vi "Motor_pwm_controle_de_posicao_3.vi"() -> ()   [LabVIEW 2018]
uses:
  <vilib>/Platform/TimedLoop/XDataNode/timing_clust.ctl
  <vilib>/Platform/TimedLoop/XDataNode/nitl_modes.ctl
  <vilib>/Platform/TimedLoop/XDataNode/wakeup.ctl
  <vilib>/Analysis/3filter.llb/Savitzky-Golay Filter (DBL).vi
  <vilib>/platform/TimedLoop/XDataNode/XDataNode.xnode
  <vilib>/Platform/TimedLoop/XDataNode/XDNodeRunTimeDep.lvlib
  <vilib>/Analysis/NI_AALBase.lvlib
panel:
  out "size(s)":i32
  out "Posições alcançadas (°)":dbl[](array[numeric])
  in  "Posições desejadas (°)":dbl[](array[numeric])
  out "Posição do motor":dbl[](graph)
  out "Aceleração":dbl[](graph)
  out "Velocidade de rotação do motor":dbl[](graph)
  out "Diferença entre a posição atual e a desejada (°)":dbl
  in  "Taxa de convergência":dbl(slide) scale=0.0..5.0
  out "Sentido de Rotação":enum16{"Horário", "Anti-Horário"}(ring)
  in  "Tab Control":enum32{"Posição", "Velocidade", "Aceleração"}(tab)
  out "Posição Acumulada":waveform(dbl)(graph)
  out "Velocidade Acumulada":waveform(dbl)(graph)
  out "Aceleração acumulada":waveform(dbl)(graph)
  in  "Frequência do PWM (Hz)":dbl
  in  "stop":bool
  in  "Iniciar controle":bool
  in  "Tensão de alimentação (V)":dbl
  # "CONTROLE DE POSI敲O DE MOTOR DC"
  # "Controle de posição por PWM desenvolvido para um motor DC simulado"
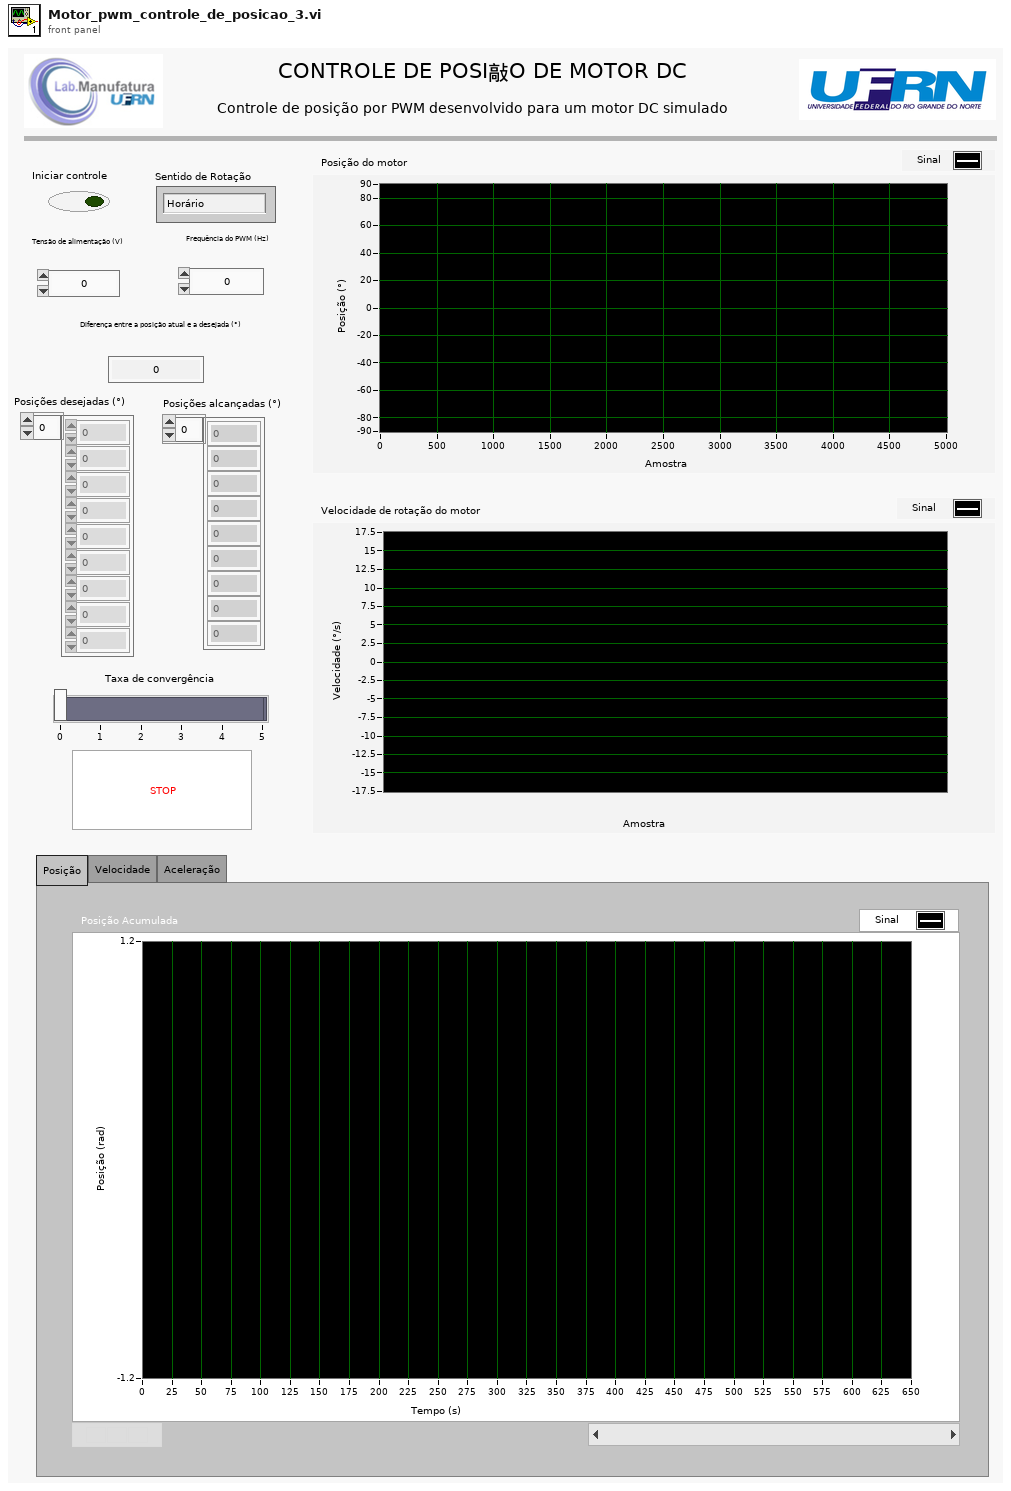
[diagram p1: front panel]
types:
  T1 = typedef "XDNodeRunTimeDep.lvlib/timing_clust.ctl" = cluster{"Expected End [f-1]":u64, "Actual End [f-1]":u64, "Finished Late? [f-1]":bool, "Expected End [i-1]":u64, "Actual End [i-1]":u64, "Finished Late? [i-1]":bool, "Expected Start [i]":u64, "Actual Start [i]":u64, "Expected Start [f]":u64, "Actual Start [f]":u64, "Source Name":string, "Structure Name":string, "Period":i64, "Deadline":i64, "Offset":i64, "Start":i64, "Priority":i32, "Timeout":i32, "Mode":T2, "Wakeup Reason":T3, "Error":errorcluster, "Source Type":string, "Secondary Source Type":string, "Global End Time":u64, "Global Start Time":u64, "Frame Duration":u64, "Iteration Duration":u64, "Assigned CPU":i32, "I/O Scan Engine Mode":u32}
  T2 = typedef "XDNodeRunTimeDep.lvlib/nitl_modes.ctl" = enum32{"No Change", "Process missed periods, maintain original phase", "Discard missed periods, maintain original phase", "Process missed periods, ignore original phase", "Discard missed periods, ignore original phase"}
  T3 = typedef "XDNodeRunTimeDep.lvlib/wakeup.ctl" = enum32{"Normal", "Aborted", "Asynchronous wakeup", "Timing source error", "Timed loop error", "Timeout"}
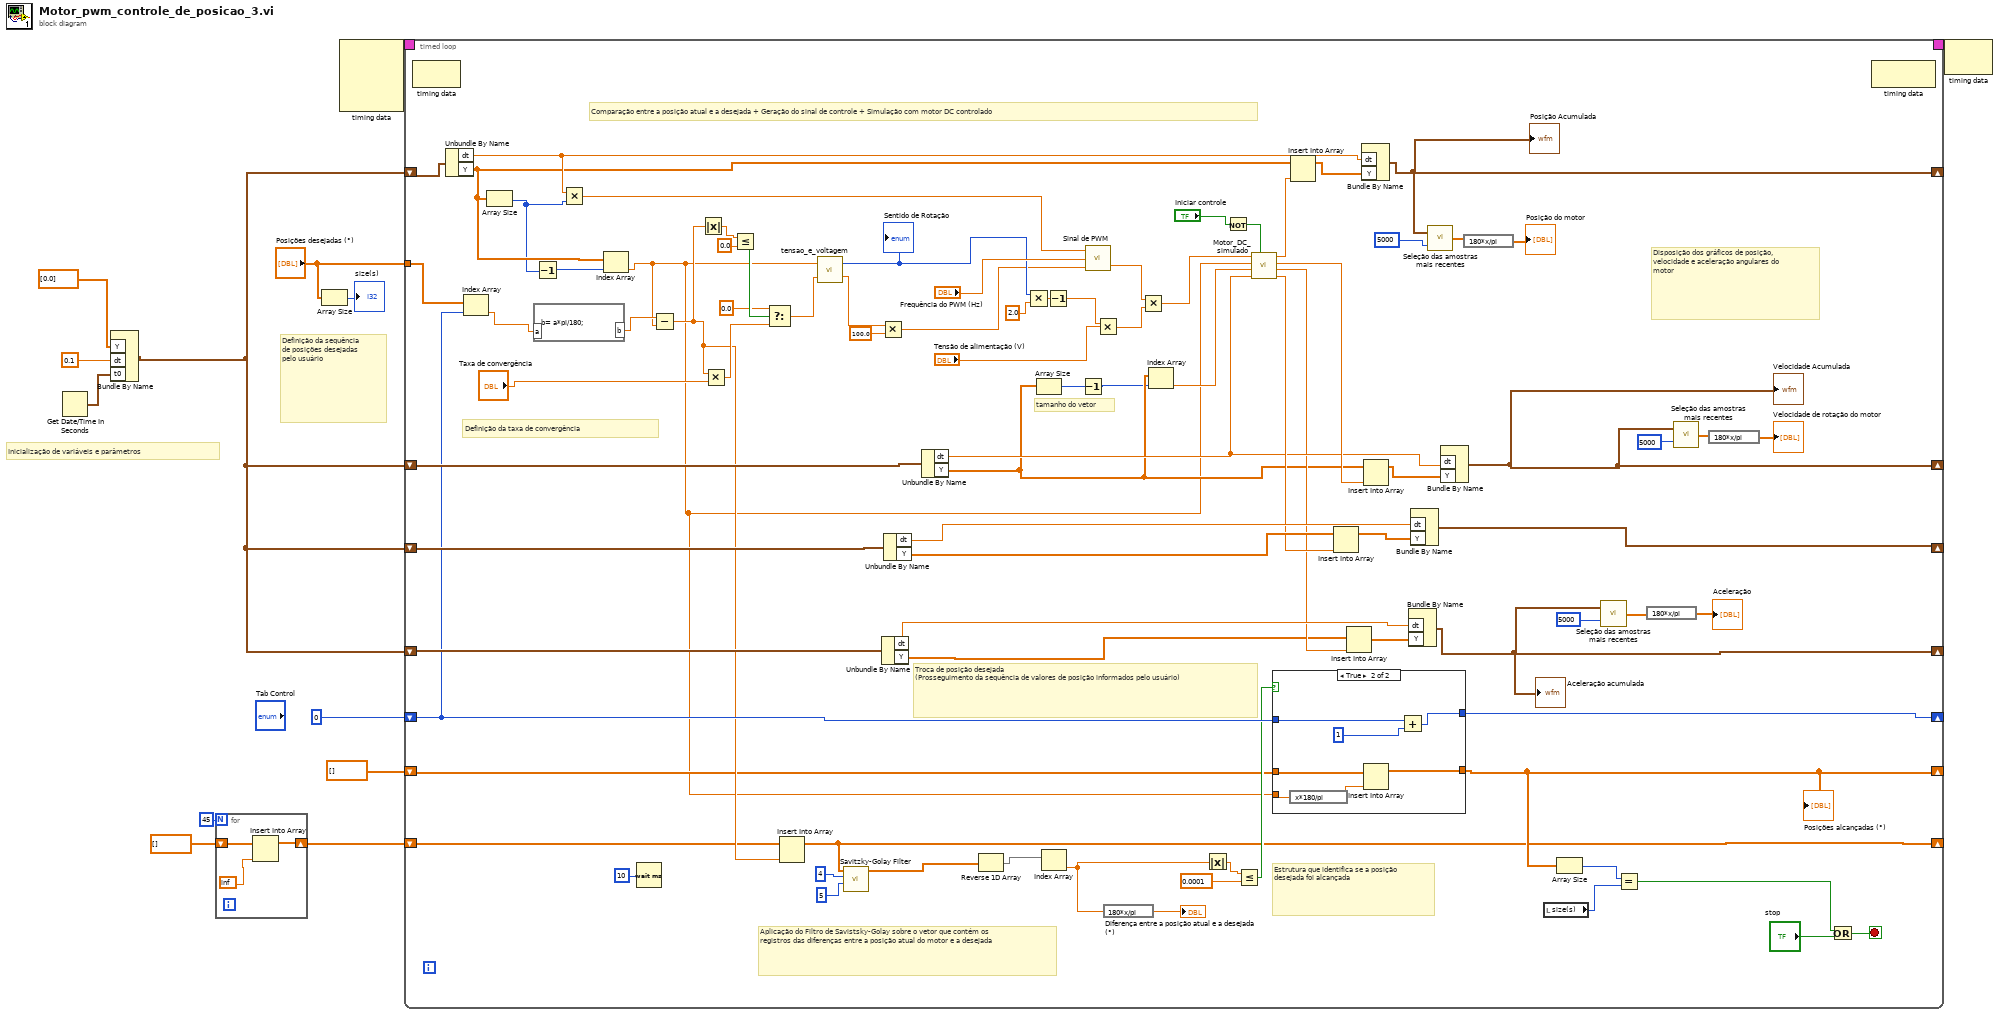
[diagram p0: block diagram]
diagram:
  # "Inicialização de variáveis e parâmetros"
  # "Definição da sequência de posições desejadas pelo usuário"
  n1 = Get Date/Time In Seconds() -> (seconds since 1Jan1904=w10:timestamp)
  n2 = Bundle By Name("Y"=dbl[] [0.0], "dt"=0.1, "t0"=w10) -> (w8:waveform(dbl))  [unwired: 1 in]
  n3 = for {
    N: 45 -> [_]
    shift-right: [w15] -> w4
    shift-left: dbl[] [] ("array") -> [w16]
    n4 = Insert Into Array(array=w16, new element=inf ("new element/subarray")) -> (w15:dbl[])  [unwired: 1 in]
  }
  n5 = Array Size(array="Posições desejadas (°)") -> (size(s)=→"size(s)":i32)
  n6 = node-c288() -> (w13:T1)  [unwired: 4 in]
  n7 = timed-loop {
    shift-right: [w99] -> _
    shift-left: w8 -> [w100]
    shift-right: [w48] -> _
    shift-left: w8 -> [w102]
    shift-right: [w98] -> _
    shift-left: w8 -> [w101]
    shift-right: [w96] -> _
    shift-left: w8 -> [w97]
    timing: w13 -> [_]
    timing-out: [_] -> w12
    shift-right: [w44] -> _
    shift-left: 0 ("index") -> [w45]
    tunnel: "Posições desejadas (°)" -> [w43]
    shift-right: [w26] -> _
    shift-left: w4 -> [w39]
    shift-right: [w30] -> _
    shift-left: dbl[] [] ("array") -> [w34]
    stop <- w32 stop-if-true
    # "Disposição dos gráficos de posição, velocidade e aceleração angulares do motor"
    # "Estrutura que identifica se a posição desejada foi alcançada"
    # "Troca de posição desejada\n(Prosseguimento da sequência de valores de posição informados pelo usuário)"
    # "Aplicação do Filtro de Savistsky-Golay sobre o vetor que contém os registros das diferenças entre a posição atual do motor e a desejada"
    # "Comparação entre a posição atual e a desejada + Geração do sinal de controle + Simulação com motor DC controlado"
    # "Definição da taxa de convergência"
    # "tamanho do vetor"
    n8 = node-c288() -> ()  [unwired: 1 in, 1 out]
    n9 = Unbundle By Name(w100) -> ("dt"=w67:dbl, "Y"=w65:dbl[])
    n10 = Index Array(array=w43, index=w45) -> (element=w42:dbl)
    n11 = Array Size(array=w65) -> (size(s)=w49:i32)
    n12 = formula code="b= a*pi/180;"("a"=w42) -> ("b"=w62:dbl)
    n13 = Decrement(x=w49) -> (x-1=w66:i32)
    n14 = Multiply(x=w67, y=w49) -> (x*y=w63:dbl)
    n15 = Index Array(array=w65, index=w66) -> (element=w33:dbl)
    n16 = Wait (ms)(milliseconds to wait=u32 10) -> ()  [unwired: 1 out]
    n17 = Subtract(x=w62, y=w33) -> (x-y=w40:dbl)
    n18 = Absolute Value(x=w40) -> (abs(x)=w57:dbl)
    n19 = Multiply(x=w40, y="Taxa de convergência") -> (x*y=w54:dbl)
    n20 = Less Or Equal?(x=w57, y=0.0) -> (x <= y?=w55:bool)
    n21 = Select(t=0.0, s=w55, f=w54) -> (s? t:f=w52:dbl)
    n22 = Insert Into Array(array=w39, new element=w40) -> (w26:dbl[])  [unwired: 1 in]
    n23 = call "tensao_e_voltagem.vi"("T"=w52, "th"=w33) -> ("Duty Cycle"=w60:dbl, "Sentido"=w64:enum16{"Horário", "Anti-Horário"})
    "Sentido de Rotação" <- w64
    n24 = call-poly <vilib>:"Savitzky-Golay Filter.vi"("polynomial order"=5 ("side points"), "side points"=4, "X"=w26) -> ("Filtered X"=w25:dbl[])  [unwired: 7 in, 1 out]
    n25 = Multiply(x=w60, y=100.0) -> (x*y=w58:dbl)
    n26 = Unbundle By Name(w97) -> ("dt"=w74:dbl, "Y"=w71:dbl[])
    n27 = Unbundle By Name(w101) -> ("dt"=w91:dbl, "Y"=w93:dbl[])
    n28 = Unbundle By Name(w102) -> ("dt"=w77:dbl, "Y"=w70:dbl[])
    n29 = Reverse 1D Array(array=w25) -> (reversed array=w36:dbl[])
    n30 = Multiply(x=w64, y=2.0) -> (x*y=w81:dbl)
    n31 = Array Size(array=w70) -> (size(s)=w69:i32)
    n32 = Index Array(array=w36) -> (element=w17:dbl)  [unwired: 1 in]
    n33 = Decrement(x=w81) -> (x-1=w79:dbl)
    n34 = Decrement(x=w69) -> (x-1=w68:i32)
    n35 = call "Sinal de PWM.vi"("duty cycle"=w58, "Frequência do PWM"="Frequência do PWM (Hz)", "Tempo atual"=w63) -> ("Resultado numérico"=w86:dbl)  [unwired: 1 out]
    n36 = Multiply(x=w79, y="Tensão de alimentação (V)") -> (x*y=w78:dbl)
    n37 = expression code="180*x/pi"(w17) -> (→"Diferença entre a posição atual e a desejada (°)":dbl)
    n38 = Multiply(x=w86, y=w78) -> (x*y=w85:dbl)
    n39 = Index Array(array=w70, index=w68) -> (element=w76:dbl)
    n40 = Absolute Value(x=w17) -> (abs(x)=w47:dbl)
    n41 = Not(x="Iniciar controle") -> (.not. x?=w51:bool)
    n42 = Less Or Equal?(x=w47, y=0.0001) -> (x <= y?=w41:bool)
    n43 = call "Motor_DC_simulado.vi"("Initialize"=w51, "dt"=w77, "Velocidade anterior"=w76, "Posiçao anterior"=w33, "DC_Vin"=w85) -> ("Tensão fornecida ao motor"=w90:dbl, "Aceleração"=w73:dbl, "Velocidade"=w89:dbl, "Posição"=w88:dbl)  [unwired: 2 in]
    n44 = case shown="True" w41 {
      tunnel: w45 -> [w104 w110]
      tunnel: [w104 w109] -> w44
      tunnel: w34 -> [w103 w108]
      tunnel: w33 -> [_ w106]
      tunnel: [w103 w107] -> w30
      frame False {
      }
      frame True {
        n45 = expression code="x*180/pi"(w106) -> (w105:dbl)
        n46 = Insert Into Array(array=w108, new element=w105) -> (w107:dbl[])  [unwired: 1 in]
        n47 = Add(x=w110, y=1 ("index")) -> (x+y=w109:i32)
      }
    }
    "Posições alcançadas (°)" <- w30
    n48 = Insert Into Array(array=w65, new element=w88) -> (w95:dbl[])  [unwired: 1 in]
    n49 = Insert Into Array(array=w93, new element=w90) -> (w92:dbl[])  [unwired: 1 in]
    n50 = Insert Into Array(array=w71, new element=w73) -> (w75:dbl[])  [unwired: 1 in]
    n51 = Bundle By Name("dt"=w67, "Y"=w95) -> (w99:waveform(dbl))  [unwired: 1 in]
    "Posição Acumulada" <- w99
    n52 = Insert Into Array(array=w70, new element=w89) -> (w94:dbl[])  [unwired: 1 in]
    n53 = Bundle By Name("dt"=w74, "Y"=w75) -> (w96:waveform(dbl))  [unwired: 1 in]
    "Aceleração acumulada" <- w96
    n54 = Bundle By Name("dt"=w91, "Y"=w92) -> (w98:waveform(dbl))  [unwired: 1 in]
    n55 = call "Seleção das amostras mais recentes.vi"("Número de amostras no gráfico"=5000, "Vetor de entrada"=w99) -> ("Amostras do gráfico"=w23:dbl[])
    n56 = Bundle By Name("dt"=w77, "Y"=w94) -> (w48:waveform(dbl))  [unwired: 1 in]
    "Velocidade Acumulada" <- w48
    n57 = expression code="180*x/pi"(w23) -> (→"Posição do motor":dbl[])
    n58 = local read "size(s)"() -> (w29:i32)
    n59 = Array Size(array=w30) -> (size(s)=w28:i32)
    n60 = call "Seleção das amostras mais recentes.vi"("Número de amostras no gráfico"=5000 ("Número de amostras no gráfico 2"), "Vetor de entrada"=w96) -> ("Amostras do gráfico"=w20:dbl[])
    n61 = Equal?(x=w28, y=w29) -> (x = y?=w27:bool)
    n62 = expression code="180*x/pi"(w20) -> (→"Aceleração":dbl[])
    n63 = call "Seleção das amostras mais recentes.vi"("Número de amostras no gráfico"=5000 ("Número de amostras no gráfico 2"), "Vetor de entrada"=w48) -> ("Amostras do gráfico"=w22:dbl[])
    n64 = expression code="180*x/pi"(w22) -> (→"Velocidade de rotação do motor":dbl[])
    n65 = Or(x=w27, y="stop") -> (x .or. y?=w32:bool)
    n66 = node-c288() -> ()  [unwired: 1 in, 1 out]
  }
  n67 = node-c288(w12) -> ()  [unwired: 1 out]
